vi "Actual Replot.vi"(8 "error in (no error)":errorcluster, 11 "XY WFRM Plot in":refnum<class "XY WFRM Plot.lvclass">) -> (0 "error out":errorcluster, 3 "XY WFRM Plot out":refnum<class "XY WFRM Plot.lvclass">)   [LabVIEW 2020, in "XY WFRM Plot.lvclass"]
uses:
  XY WFRM Plot.lvclass
  opt/github/LabActor/Plots/Plot/Plot.lvclass
  Plot/Plot.lvclass/Plot.ctl
  XY WFRM Plot.lvclass/XY WFRM Plot.ctl
  8cb32180-7abd-4b27-afcb-bbd739cf6f07.vi
  e6847e96-357f-421f-be23-6c38e145b2ce.vi
  c5e1e698-5171-48f6-a2a7-0a8aaa819dda.vi
  372697b9-8762-4fc7-8ff0-8d62db81c817.vi
  27d2bad1-82f0-4063-802e-88bb5171f6f1.vi
  Plot/Read Files.vi
  8cb32180-7abd-4b27-afcb-bbd739cf6f07.vi/668a06be-d8be-4049-82ee-33f1cdaacdc4.vi
  8cb32180-7abd-4b27-afcb-bbd739cf6f07.vi/2c6de516-1d23-4c23-bfc5-564dc8149620.vi
  e6847e96-357f-421f-be23-6c38e145b2ce.vi/0532bd49-aff3-45ad-9cc0-a13f982e0e17.vi
  e6847e96-357f-421f-be23-6c38e145b2ce.vi/724fb671-963e-4042-b130-e72c76e88fd9.vi
  <vilib>/Utility/error.llb/Clear Errors.vi
  372697b9-8762-4fc7-8ff0-8d62db81c817.vi/c0c8f4eb-f5dc-43a3-9fd2-6fe82153b517.vi
  372697b9-8762-4fc7-8ff0-8d62db81c817.vi/d9f28dd1-57bc-437c-abf9-381ead6ef493.vi
  8cb32180-7abd-4b27-afcb-bbd739cf6f07.vi/668a06be-d8be-4049-82ee-33f1cdaacdc4.vi/f32759e9-418f-4dd9-99d9-892840a9754a.vi
  e6847e96-357f-421f-be23-6c38e145b2ce.vi/0532bd49-aff3-45ad-9cc0-a13f982e0e17.vi/1bcf6eca-5e38-4694-9c6b-5dcad1ef6d61.vi
  372697b9-8762-4fc7-8ff0-8d62db81c817.vi/c0c8f4eb-f5dc-43a3-9fd2-6fe82153b517.vi/579b74a7-738b-41b6-a2c9-a5c73b95a491.vi
  NHMFL_Core/Libraries/File/TDMS/TDMS Open Err Check.vi
  NHMFL_Core/Libraries/File/Get TDMS channel info.vi
  <vilib>/measure/maresamp.llb/Resample Waveforms (single shot).vi
  <vilib>/measure/maresamp.llb/Resample Waveform (single shot).vi
  NHMFL_Core/Libraries/Utilities/Waveform/AvrgDecimate.vi
  NHMFL_Core/Libraries/Utilities/Waveform/MaxMinDecimate.vi
  Plot/Plot.lvclass
  <vilib>/ErrorRing/Error Ring.xnode
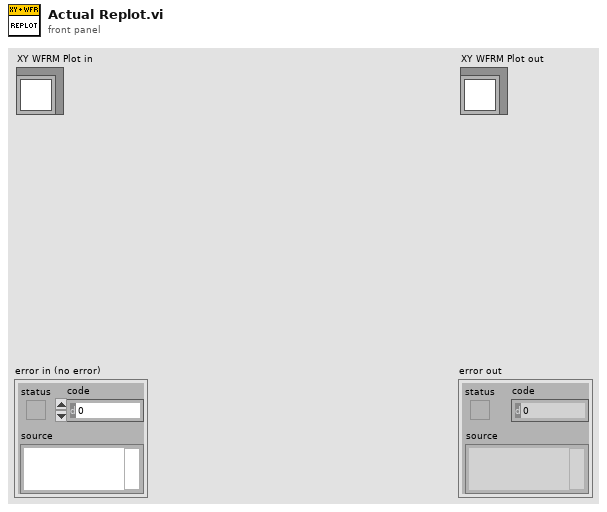
[diagram p1: front panel]
types:
  T1 = typedef "Plot types.ctl" = enum16{"Waveform Plot", "XY Plot", "Full XY"}
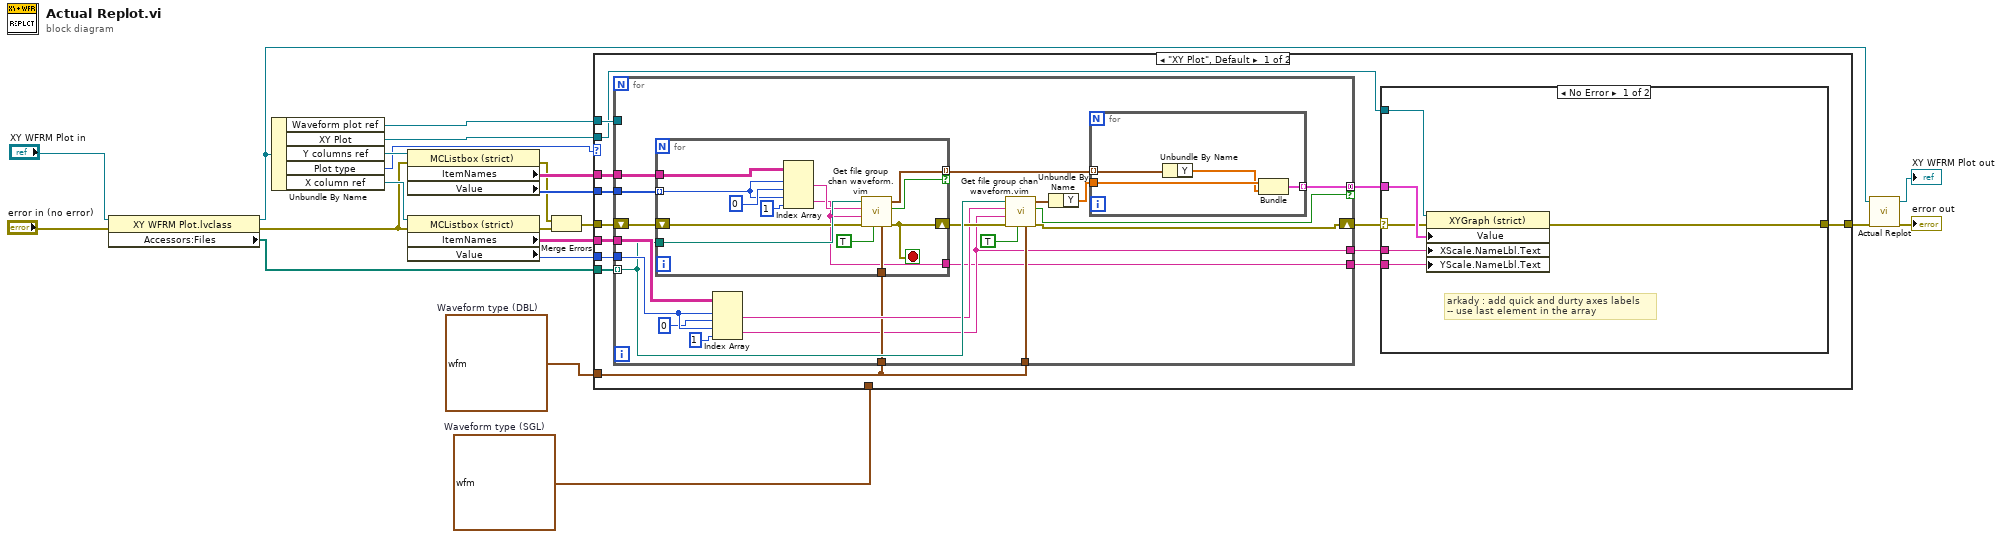
[diagram p0: block diagram]
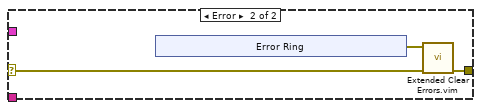
[diagram p2: hidden frame]
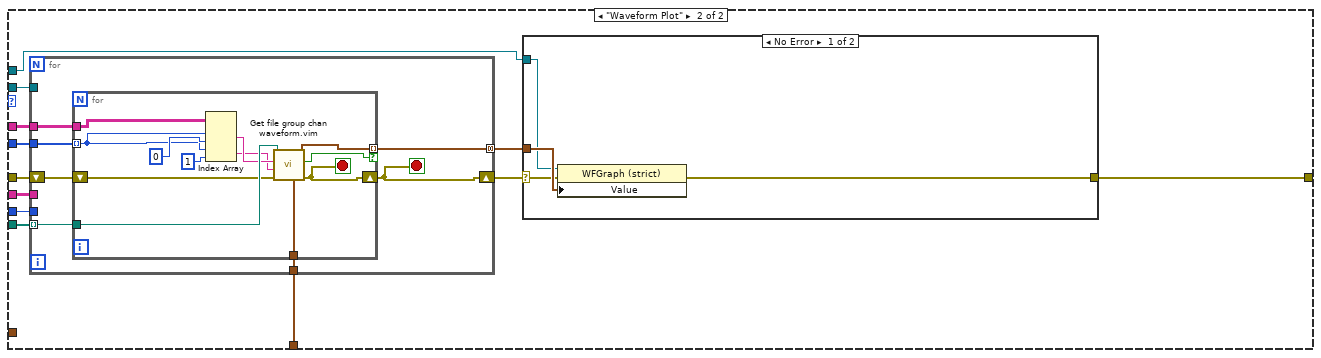
[diagram p3: hidden frame]
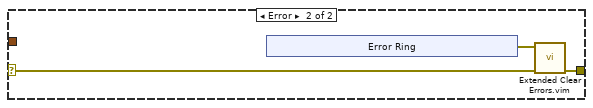
[diagram p4: hidden frame]
diagram:
  w1 = waveform(sgl) {"t0"=timestamp(0 s since 1904-01-01), "dt"=1.0, "Y"=[]}  # Waveform type (SGL)
  w2 = waveform(dbl) {"t0"=timestamp(0 s since 1904-01-01), "dt"=1.0, "Y"=[]}  # Waveform type (DBL)
  n1 = property class="XY WFRM Plot.lvclass"(reference="XY WFRM Plot in", error in="error in (no error)") -> (reference out=w4:refnum<class "XY WFRM Plot.lvclass">, error out=w11:errorcluster, "Accessors:Files"=w18:path[])
  n2 = Unbundle By Name(w4) -> ("Waveform plot ref"=w13:refnum<vi>, "XY Plot"=w14:refnum<vi>, "Y columns ref"=w21:refnum<vi>, "Plot type"=w10:T1, "X column ref"=w17:refnum<vi>)
  n3 = property class="MCListbox (strict)"(reference=w21, error in=w11) -> (error out=w9:errorcluster, "ItemNames"=w20:string[][], "Value"=w19:i32[])  [unwired: 1 out]
  n4 = property class="MCListbox (strict)"(reference=w17, error in=w11) -> (error out=w8:errorcluster, "ItemNames"=w15:string[][], "Value"=w16:i32)  [unwired: 1 out]
  n5 = Merge Errors(w9, w8) -> (w7:errorcluster)
  n6 = case shown="\"XY Plot\", Default" w10 {
    tunnel: w20 -> [w36 w96]
    tunnel: w19 -> [w35 w95]
    tunnel: w18 -> [w34 w94]
    tunnel: w16 -> [w33 w93]
    tunnel: w15 -> [w32 w92]
    tunnel: w14 -> [w28 w91]
    tunnel: w13 -> [w31 w88]
    tunnel: [w29 w89] -> w6
    tunnel: w7 -> [w27 w87]
    tunnel: w2 -> [w25 _]
    tunnel: w1 -> [_ w85]
    frame "XY Plot", Default {
      n7 = for {
        tunnel: w36 -> [w67]
        tunnel: w35 -> [w66]
        tunnel: w34 -> [w62] mode=indexing
        shift-right: [w53] -> w26
        shift-left: w27 -> [w65]
        tunnel: w33 -> [w64]
        tunnel: w32 -> [w63]
        tunnel: w31 -> [_]
        tunnel: [w54] -> w30 mode=concatenating if=w52
        tunnel: w25 -> [w50]
        tunnel: w25 -> [w49]
        tunnel: [w48] -> w24
        tunnel: [w47] -> w23
        n8 = for {
          tunnel: w67 -> [w84]
          tunnel: w66 -> [w82] mode=indexing
          tunnel: w62 -> [w80]
          shift-right: [w74] -> w60
          shift-left: w65 -> [w78]
          tunnel: [w77] -> w61 mode=indexing if=w76
          tunnel: w49 -> [w73]
          tunnel: [w72] -> w47
          stop <- w74 stop-if-true
          n9 = Index Array(array=w84, index (row) #1=w82, index (col) #1=0 ("disabled index (col)"), index (row) #2=w82, index (col) #2=1 ("disabled index (col)")) -> (element #1=w79:string, element #2=w72:string)
          n10 = call "Get file group chan waveform.vim"("Waveform type"=w73, "Clear missing ch err"=TRUE, "Error In"=w78, "Channel"=w72, "Group"=w79, "File"=w80) -> ("Error Out"=w74:errorcluster, "Valid WFRM"=w76:bool, "Waveform"=w77:waveform(dbl))  [unwired: 3 in]
        }
        n11 = Index Array(array=w63, index (row) #1=w64, index (col) #1=0 ("index (col)"), index (row) #2=w64, index (col) #2=1 ("index (col)")) -> (element #1=w57:string, element #2=w48:string)
        n12 = call "Get file group chan waveform.vim"("Waveform type"=w50, "Clear missing ch err"=TRUE, "Error In"=w60, "Channel"=w48, "Group"=w57, "File"=w62) -> ("Error Out"=w53:errorcluster, "Valid WFRM"=w52:bool, "Waveform"=w56:waveform(dbl))  [unwired: 3 in]
        n13 = Unbundle By Name(w56) -> ("Y"=w55:dbl[])
        n14 = for {
          tunnel: w55 -> [w71]
          tunnel: w61 -> [w70] mode=indexing
          tunnel: [w68] -> w54 mode=indexing
          n15 = Unbundle By Name(w70) -> ("Y"=w69:dbl[])
          n16 = Bundle("Y"=w71, "Y"=w69) -> (w68:cluster{"Y":dbl[], "Y":dbl[]})  [unwired: 1 in]
        }
      }
      n17 = case shown="No Error" w26 {
        selector: w26 -> [w39 w44]
        tunnel: w30 -> [w42 _]
        tunnel: [w41 w43] -> w29
        tunnel: w28 -> [w40 _]
        tunnel: w24 -> [w38 _]
        tunnel: w23 -> [w37 _]
        frame No Error {
          # "arkady : add quick and durty axes labels \n-- use last element in the array"
          n18 = property class="XYGraph (strict)"(reference=w40, error in=w39, "Value"=w42, "XScale.NameLbl.Text"=w38, "YScale.NameLbl.Text"=w37) -> (error out=w41:errorcluster)  [unwired: 1 out]
        }
        frame Error {
          n19 = xnode "Error Ring"() -> ("error out"=w45:errorcluster)
          n20 = call "Extended Clear Errors.vim"("Error In"=w44, "specific error code to clear (0: all)"=w45) -> ("Error Out"=w43:errorcluster)  [unwired: 7 in, 2 out]
        }
      }
    }
    frame "Waveform Plot" {
      n21 = for {
        tunnel: w96 -> [w111]
        tunnel: w95 -> [w110]
        tunnel: w94 -> [w108] mode=indexing
        shift-right: [w106] -> w86
        shift-left: w87 -> [w109]
        tunnel: w93 -> [_]
        tunnel: w92 -> [_]
        tunnel: w91 -> [_]
        tunnel: [w107] -> w90 mode=concatenating
        tunnel: w85 -> [w105]
        stop <- w106 stop-if-true
        n22 = for {
          tunnel: w111 -> [w123]
          tunnel: w110 -> [w121] mode=indexing
          tunnel: w108 -> [w119]
          shift-right: [w113] -> w106
          shift-left: w109 -> [w116]
          tunnel: [w115] -> w107 mode=indexing if=w114
          tunnel: w105 -> [w112]
          stop <- w113 stop-if-true
          n23 = Index Array(array=w123, index (row) #1=w121, index (col) #1=0 ("disabled index (col)"), index (row) #2=w121, index (col) #2=1 ("disabled index (col)")) -> (element #1=w118:string, element #2=w117:string)
          n24 = call "Get file group chan waveform.vim"("Waveform type"=w112, "Error In"=w116, "Channel"=w117, "Group"=w118, "File"=w119) -> ("Error Out"=w113:errorcluster, "Valid WFRM"=w114:bool, "Waveform"=w115:waveform(sgl))  [unwired: 4 in]
        }
      }
      n25 = case shown="No Error" w86 {
        selector: w86 -> [w97 w102]
        tunnel: w90 -> [w100 _]
        tunnel: [w99 w103] -> w89
        tunnel: w88 -> [w98 _]
        frame No Error {
          n26 = property class="WFGraph (strict)"(reference=w98, error in=w97, "Value"=w100) -> (error out=w99:errorcluster)  [unwired: 1 out]
        }
        frame Error {
          n27 = xnode "Error Ring"() -> ("error out"=w101:errorcluster)
          n28 = call "Extended Clear Errors.vim"("Error In"=w102, "specific error code to clear (0: all)"=w101) -> ("Error Out"=w103:errorcluster)  [unwired: 7 in, 2 out]
        }
      }
    }
  }
  n29 = call-parent "Actual Replot.vi"("error in (no error)"=w6, "Plot in"=w4) -> ("error out"=→"error out":errorcluster, "Plot out"=→"XY WFRM Plot out":refnum<class "XY WFRM Plot.lvclass">)  [unwired: 8 in]
